vi "Relative Seconds.vi"(10 "Relative Seconds in":dbl format="%_19f", 11 "error in (no error)":errorcluster) -> (1 "Relative Seconds delta":dbl format="%_19f", 2 "Relative Seconds out":dbl format="%_19f", 3 "error out":errorcluster)   [LabVIEW 2015, in "Utility.lvlib"]
uses:
  Utility.lvlib
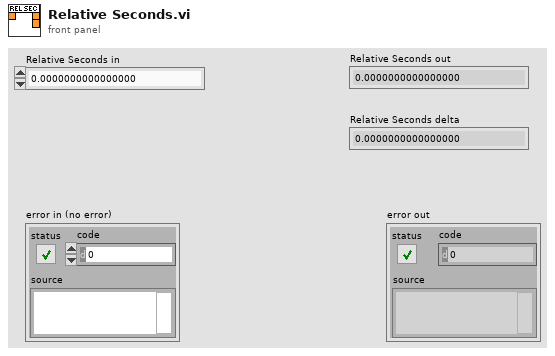
[diagram p1: front panel]
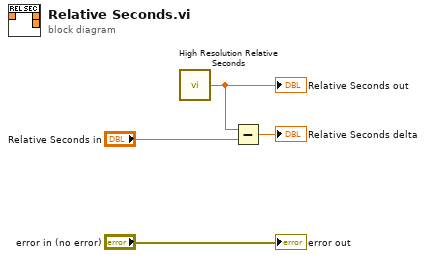
[diagram p0: block diagram]
diagram:
  n1 = call <vilib>:"High Resolution Relative Seconds.vi"() -> ("relative seconds"=w3:dbl)
  "Relative Seconds out" <- w3
  n2 = Subtract(x=w3, y="Relative Seconds in") -> (x-y=→"Relative Seconds delta":dbl)
  "error out" <- "error in (no error)"
